vi "SubVI_Extract #.vi"(5 "Extract Direction":T3(ring), 7 "Image Register Name":string="untitled", 8 "Error in":errorcluster, 9 "ROI Descriptor":T2 {"Contours"."Type" items=["No Selection", "Point", "Line", "Rectangle", "Oval", "Polygon", "Freehand Region", "Annulus", "Unused2", "Unused3", "Broken Line", "Freehand Line", "Rotated Rectangle"]}, 10 "Extract Potion":cluster{"X":i32, "Y":i32}, 11 "Image Src In":T1) -> (0 "Error out":errorcluster, 1 "ROI Descriptor out":T2 {"Contours"."Type" items=["No Selection", "Point", "Line", "Rectangle", "Oval", "Polygon", "Freehand Region", "Annulus", "Unused2", "Unused3", "Broken Line", "Freehand Line", "Rotated Rectangle"]}, 2 "Image Src Out":T1, 3 "Image Dst Out":T1)   [LabVIEW 2013]
uses:
  <vilib>/vision/Image Controls.llb/IMAQ Image.ctl
  <vilib>/vision/NI_Vision_Development_Module.lvlib
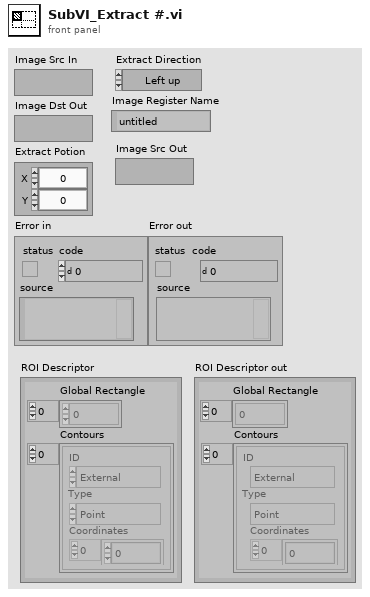
[diagram p1: front panel]
types:
  T1 = typedef "IMAQ Image.ctl" = refnum<image>
  T2 = typedef "ROI Descriptor" = cluster{"Global Rectangle":i32[], "Contours":cluster{"ID":enum32{"External", "Internal"}, "Type":u32, "Coordinates":i32[]}[]}
  T3 = enum16{"Left up", "Right up", "Left Down", "Right Down"}
  T4 = cluster{"Origin":cluster{"X":sgl, "Y":sgl}, "Angle (deg)":sgl, "Axis Reference":u32}
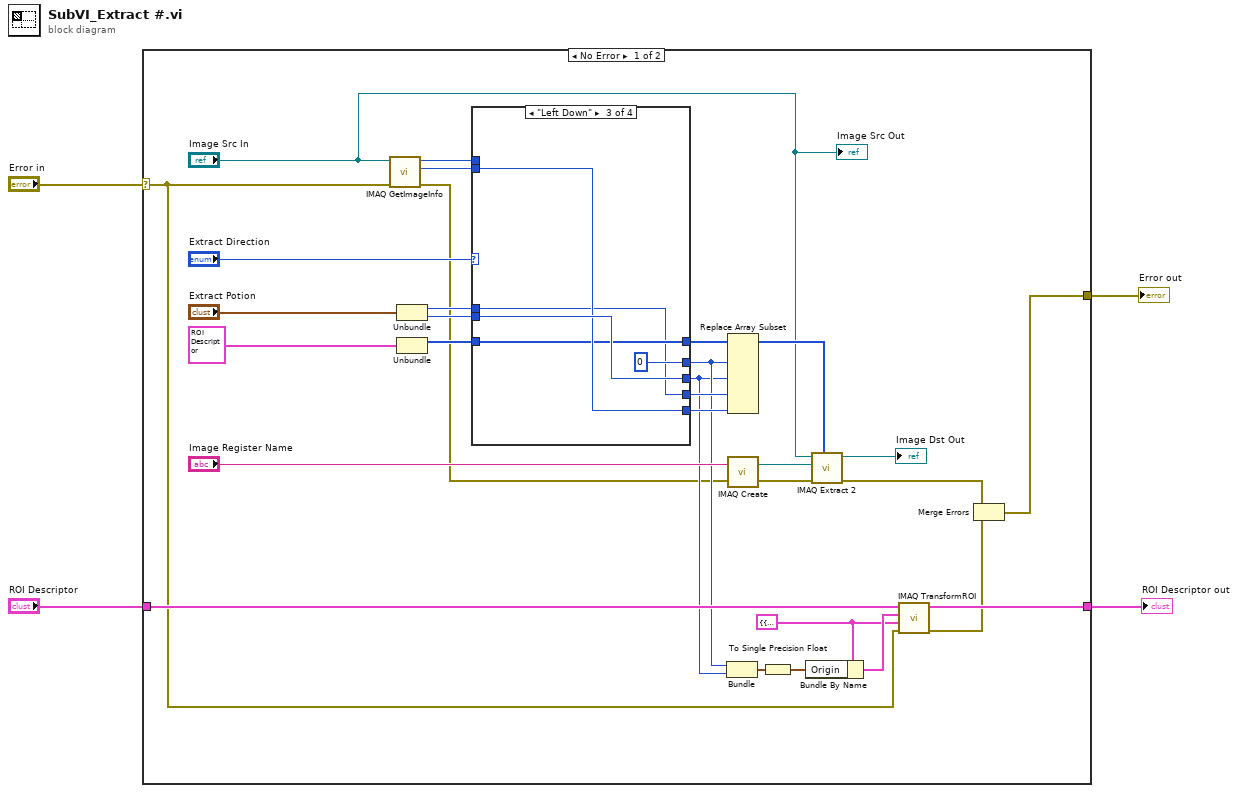
[diagram p0: block diagram]
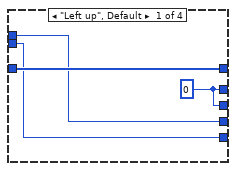
[diagram p2: hidden frame]
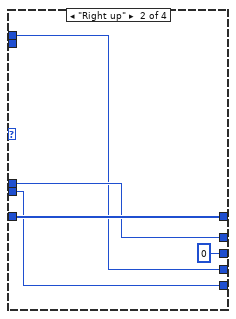
[diagram p3: hidden frame]
diagram:
  n1 = case shown="No Error" "Error in" {
    selector: "Error in" -> [w9 w55]
    tunnel: [w6 w55] -> w3
    tunnel: "ROI Descriptor" -> [w16 w54]
    tunnel: [w11 w54] -> w1
    frame No Error {
      w17 = T4 {"Origin"={"X"=0.0, "Y"=0.0}, "Angle (deg)"=0.0, "Axis Reference"=0} ("Base Reference")
      n2 = call "IMAQ GetImageInfo"("error in (no error)"=w9, "Image"="Image Src In") -> ("error out"=w10:errorcluster, "Y Resolution"=w23:i32, "X Resolution"=w24:i32)  [unwired: 2 in, 5 out]
      n3 = Unbundle("Extract Potion") -> ("X"=w29:i32, "Y"=w28:i32)
      n4 = Unbundle(T2 {"Global Rectangle"=[0, 0, 0, 0], "Contours"=[{"ID"=enum."External", "Type"=3, "Coordinates"=[0, 0, 0, 0, 0, 0]}]} ("ROI Descriptor")) -> ("Global Rectangle"=w33:i32[])  [unwired: 1 out]
      n5 = case shown="\"Left Down\"" "Extract Direction" {
        tunnel: w33 -> [w37 w43 w45 w53]
        tunnel: [w37 w43 w45 w53] -> w32
        tunnel: w29 -> [w36 w41 w44 w52]
        tunnel: w28 -> [w35 w42 w48 w51]
        tunnel: [w36 w40 w44 w50] -> w26
        tunnel: [w35 w42 w46 w49] -> w27
        tunnel: [w38 w41 0 ("X") w52] -> w15
        tunnel: w24 -> [_ w40 _ w50]
        tunnel: w23 -> [_ _ w46 w49]
        tunnel: [w38 0 ("Y") w48 w51] -> w14
        frame "Left up", Default {
          w38 = 0 ("X")
        }
        frame "Right up" {
        }
        frame "Left Down" {
        }
        frame "Right Down" {
        }
      }
      n6 = Bundle("X"=w15, "Y"=w14) -> (w13:cluster{"X":i32, "Y":i32})  [unwired: 1 in]
      n7 = Replace Array Subset(array=w32, new element #1=w15, new element #2=w14, new element #3=w26, new element #4=w27) -> (w25:i32[])  [unwired: 4 in]
      n8 = call "IMAQ Create"("Image Name"="Image Register Name", "error in (no error)"=w10) -> ("New Image"=w21:T1, "error out"=w19:errorcluster)  [unwired: 3 in]
      n9 = To Single Precision Float(number=w13) -> (single precision float=w12:cluster{"X":sgl, "Y":sgl})
      n10 = Bundle By Name(cluster=w17, "Origin"=w12) -> (w18:T4)
      n11 = call "IMAQ Extract 2"("Optional Rectangle"=w25, "error in (no error)"=w19, "Image Dst"=w21, "Image Src"="Image Src In") -> ("error out"=w8:errorcluster, "Image Dst Out"=→"Image Dst Out":T1)  [unwired: 6 in]
      n12 = call "IMAQ TransformROI"("error in (no error)"=w9, "New Reference"=w17, "Base Reference"=w18, "ROI Descriptor"=w16) -> ("error out"=w7:errorcluster, "ROI Descriptor out"=w11:T2)  [unwired: 6 in]
      n13 = Merge Errors(w8, w7) -> (w6:errorcluster)
      "Image Src Out" <- "Image Src In"
    }
    frame Error {
    }
  }
  "Error out" <- w3
  "ROI Descriptor out" <- w1
